vi "UHR-Fleezers Control (host) - 12.6.vi"() -> ()   [LabVIEW 2012] (continued)
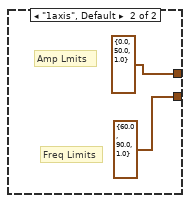
[diagram p2: hidden frame]
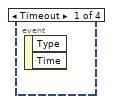
[diagram p3: hidden frame]
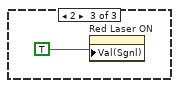
[diagram p6: hidden frame]
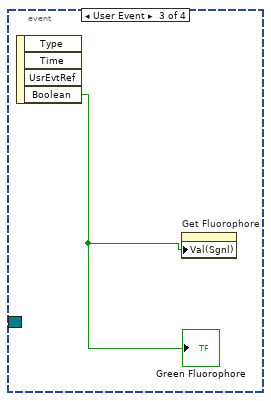
[diagram p7: hidden frame]
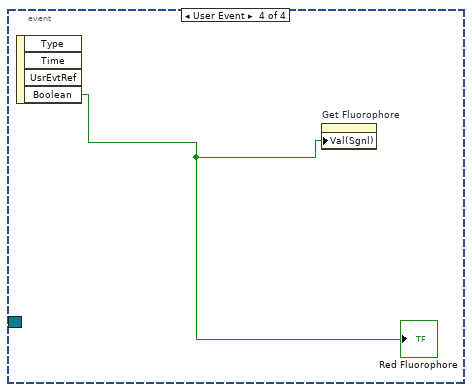
[diagram p8: hidden frame]
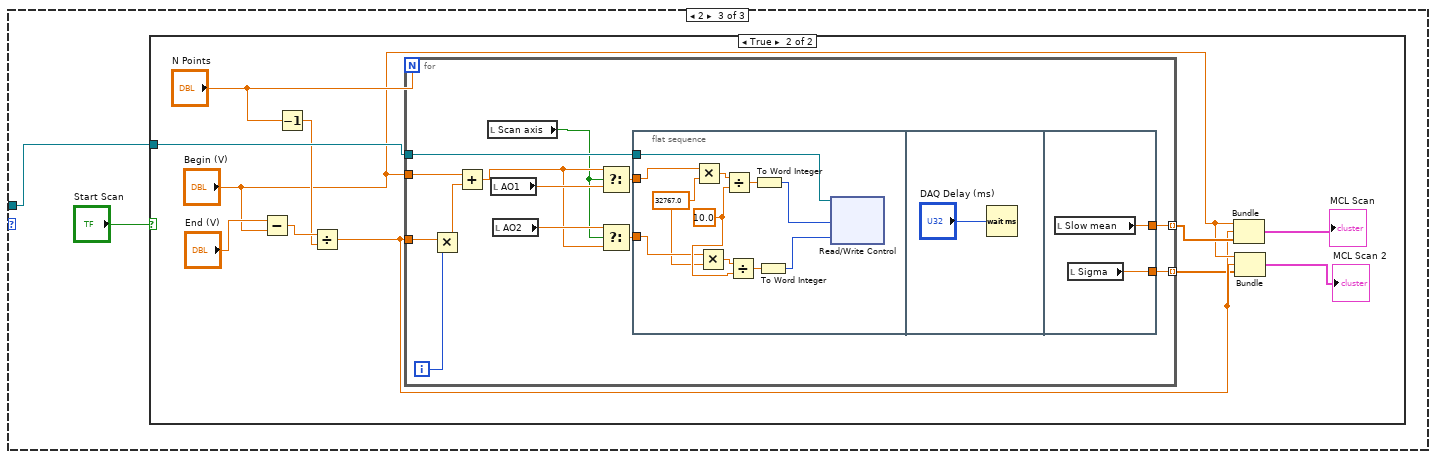
[diagram p10: hidden frame]
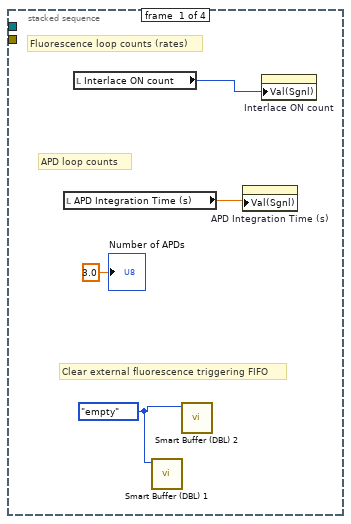
[diagram p12: hidden frame]
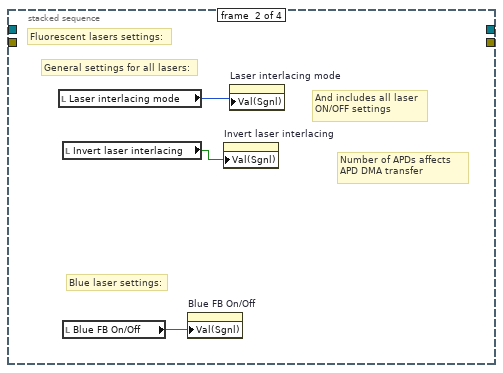
[diagram p13: hidden frame]
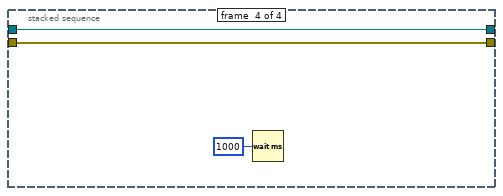
[diagram p14: hidden frame]
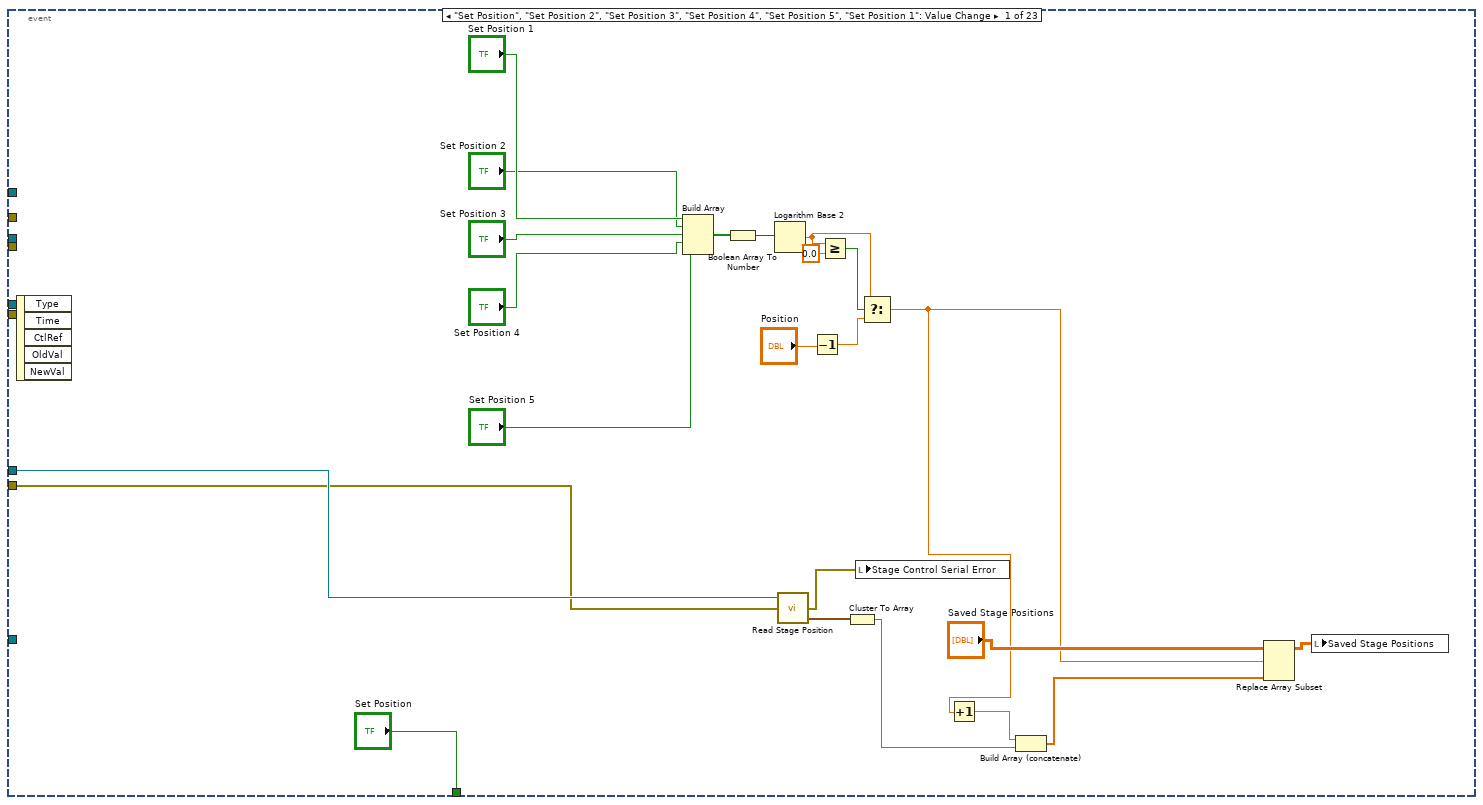
[diagram p16: hidden frame]
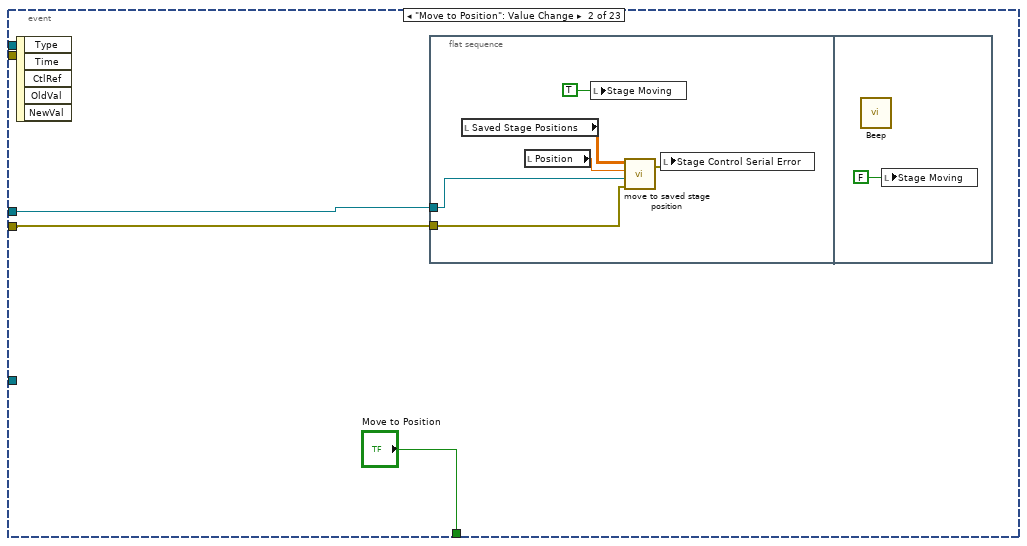
[diagram p17: hidden frame]
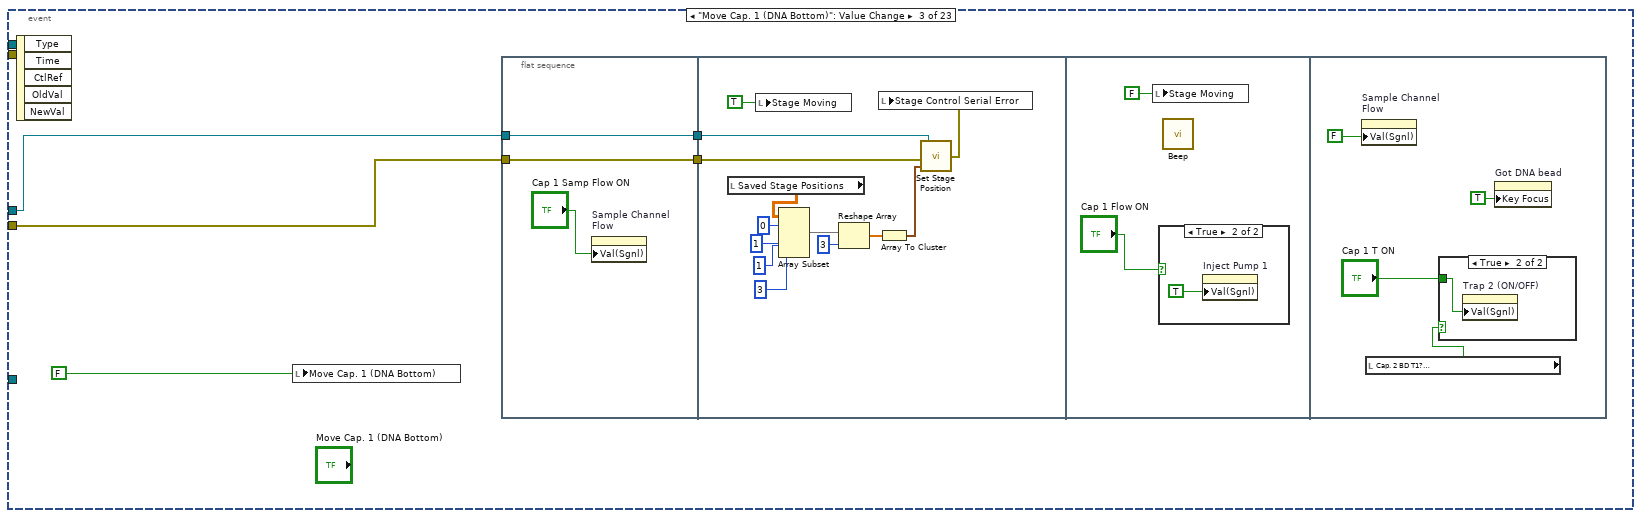
[diagram p18: hidden frame]
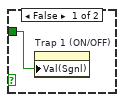
[diagram p20: hidden frame]
          n3238 = Divide(x=w5129, y=10.0) -> (x/y=w5130:dbl)
          n3239 = To Word Integer(number=w5135) -> (16bit integer=w5127:i16)
          n3240 = To Word Integer(number=w5130) -> (16bit integer=w5126:i16)
          n3241 = Divide(x=w5138, y=i64 1000) -> (x/y=w5109:dbl)
          n3242 = Multiply(x=w5109, y=w5139) -> (x*y=w5120:dbl)
          n3243 = Multiply(x="Osc. freq. (Hz) 2", y=6.283185307179586) -> (x*y=w5121:dbl)
          n3244 = Multiply(x=w5121, y=w5120) -> (x*y=w5119:dbl)
          n3245 = Sine(x=w5119) -> (sin(x)=w5118:dbl)
          n3246 = Multiply(x=w5118, y="Osc. amp. (V)") -> (x*y=w5116:dbl)
          n3247 = Add(x=w5116, y="Osc. center (V)") -> (x+y=w5114:dbl)
          n3248 = Divide(x=w5114, y=10.0) -> (x/y=w5112:dbl)
          n3249 = Multiply(x=w5112, y=32767.0) -> (x*y=w5107:dbl)
          n3250 = Select(t=w5107, s="Scan axis", f=w5127) -> (s? t:f=w5125:dbl)
          n3251 = Select(t=w5126, s="Scan axis", f=w5107) -> (s? t:f=w5124:dbl)
          n3252 = local read "MCL Mode"() -> (w5106:u16)
          n3253 = Not Equal?(x=w5106, y=u16 1) -> (x != y?=w5103:bool)
          n3254 = local read "Stop All"() -> (w5104:bool)
          n3255 = xnode "Read/Write Control"("FPGA VI Reference In"=w5140, "AO1"=w5125, "AO2"=w5124) -> ()  [unwired: 1 in, 2 out]
          n3256 = Compound Arithmetic op=OR(w5104, w5103) -> (w5102:bool)
          n3257 = node-c288() -> ()  [unwired: 2 out]
        }
        n3258 = node-c288(w5100) -> ()  [unwired: 1 out]
      }
      frame 2 {
        n3259 = case shown="True" "Start Scan" {
          tunnel: w5146 -> [_ w5158]
          frame False {
          }
          frame True {
            n3260 = Subtract(x="End (V)", y="Begin (V)") -> (x-y=w5154:dbl)
            n3261 = Decrement(x="N Points") -> (x-1=w5153:dbl)
            n3262 = Divide(x=w5154, y=w5153) -> (x/y=w5151:dbl)
            n3263 = for {
              N: "N Points" -> [_]
              tunnel: "Begin (V)" -> [w5171]
              tunnel: w5158 -> [w5163]
              tunnel: [w5162] -> w5157 mode=indexing
              tunnel: w5151 -> [w5161]
              tunnel: [w5159] -> w5150 mode=indexing
              i -> [w5170]
              n3264 = Multiply(x=w5161, y=w5170) -> (x*y=w5169:dbl)
              n3265 = Add(x=w5171, y=w5169) -> (x+y=w5166:dbl)
              n3266 = local read "Scan axis"() -> (w5160:bool)
              n3267 = local read "AO1"() -> (w5168:dbl)
              n3268 = local read "AO2"() -> (w5167:dbl)
              n3269 = Select(t=w5166, s=w5160, f=w5168) -> (s? t:f=w5165:dbl)
              n3270 = Select(t=w5167, s=w5160, f=w5166) -> (s? t:f=w5164:dbl)
              n3271 = flat-sequence {
                tunnel: w5165 -> [w5175]
                tunnel: w5164 -> [w5174]
                tunnel: w5163 -> [w5172]
                tunnel: [w5185] -> w5162
                tunnel: [w5184] -> w5159
                frame #0 {
                  w5178 = 10.0 ("y")
                  w5173 = 32767.0 ("y")
                  n3272 = Multiply(x=w5175, y=w5173) -> (x*y=w5181:dbl)
                  n3273 = Multiply(x=w5174, y=w5173) -> (x*y=w5179:dbl)
                  n3274 = Divide(x=w5181, y=w5178) -> (x/y=w5182:dbl)
                  n3275 = Divide(x=w5179, y=w5178) -> (x/y=w5180:dbl)
                  n3276 = To Word Integer(number=w5182) -> (16bit integer=w5176:i16)
                  n3277 = To Word Integer(number=w5180) -> (16bit integer=w5177:i16)
                  n3278 = xnode "Read/Write Control"("FPGA VI Reference In"=w5172, "AO1"=w5176, "AO2"=w5177) -> ()  [unwired: 1 in, 2 out]
                }
                frame #1 {
                  n3279 = Wait (ms)(milliseconds to wait="DAQ Delay (ms)") -> ()  [unwired: 1 out]
                }
                frame #2 {
                  n3280 = local read "Slow mean"() -> (w5185:dbl)
                  n3281 = local read "Sigma"() -> (w5184:dbl)
                }
              }
            }
            n3282 = Bundle("Begin (V)"="Begin (V)", w5151, w5157) -> (→"MCL Scan":cluster{"Begin (V)":dbl, dbl, dbl[]})  [unwired: 1 out]
            n3283 = Bundle("Begin (V)"="Begin (V)", w5151, w5150) -> (→"MCL Scan 2":cluster{"Begin (V)":dbl, dbl, dbl[]})  [unwired: 1 out]
          }
        }
      }
    }
    n3284 = local read "Stop All"() -> (w5095:bool)
    n3285 = node-c288() -> ()  [unwired: 2 out]
  }
  n3286 = node-c288(w9) -> ()  [unwired: 1 out]
  n3287 = node-c288(w125) -> ()  [unwired: 1 out]
  n3288 = node-c288(w127) -> ()  [unwired: 1 out]
  n3289 = property on="Saved trap pos" class="WFGraph (strict)"("Visible"=FALSE) -> ()  [unwired: 2 in, 2 out]
  n3290 = property on="Trap Delta Graph" class="WFGraph (strict)"("Visible"=TRUE) -> ()  [unwired: 2 in, 2 out]
  n3291 = node-c288(w112) -> ()  [unwired: 1 out]
  n3292 = local write "Trap pos"(FALSE ("Trap pos")) -> ()
  n3293 = disable-structure shown="Disabled" {
    disable-tunnel: w116 -> [w5187 _]
    disable-tunnel: w115 -> [w5186 _]
    frame Disabled {
      n3294 = VISA Close(VISA resource name=w5187, error in (no error)=w5186) -> (error out=w5188:errorcluster)
      n3295 = call <vilib>:"Simple Error Handler.vi"("error in (no error)"=w5188) -> ()  [unwired: 1 in, 8 out]
    }
    frame Enabled {
    }
  }
  n3296 = node-c288(w123) -> ()  [unwired: 1 out]
  n3297 = node-c288(w198) -> ()  [unwired: 1 out]
  n3298 = flat-sequence {
    tunnel: w289 -> [w5192]
    tunnel: w291 -> [w5193]
    tunnel: [w5191] -> w270
    tunnel: [w5190] -> w269
    tunnel: w254 -> [_]
    tunnel: w206 -> [_]
    tunnel: w129 -> [_]
    tunnel: w270 -> [w5194]
    tunnel: w269 -> [w5195]
    frame #0 {
      w5189 = FALSE ("AI to FIFO")
      n3299 = xnode "Read/Write Control"("FPGA VI Reference In"=w5193, "error in"=w5192, "AI to FIFO"=w5189, "APD to FIFO"=w5189) -> ("FPGA VI Reference Out"=w5191:T20, "error out"=w5190:errorcluster)
    }
    frame #1 {
      n3300 = xnode "Close FPGA VI Reference"("FPGA VI Reference In"=w5194, "error in"=w5195) -> ("error out"=→"error out":errorcluster)
    }
  }
